vi "Raw Data Send Next Chunk.vi"(8 "error in (no error)":errorcluster, 10 "trimmed string":string, 11 "Network Info":T1 {"Last Comm Time" format="%<%H:%M:%S%3u\n%Y/%m/%d>T"; "Remote Port" format="%.0x"}) -> (0 "error out":errorcluster, 3 "Network Info Out":T1 {"Last Comm Time" format="%<%H:%M:%S%3u\n%Y/%m/%d>T"; "Remote Port" format="%.0x"})   [LabVIEW 2023]
doc: "Author: Scott Hannahs <sth@magnet.fsu.edu>\nCopyright 2018 Florida State University, All rights reserved."
uses:
  RT Controls/Network Info.ctl
  RT Controls/RT System Auth Level.ctl
  TCP Functions/TCP Write Length and Data (2D Array DBL).vi
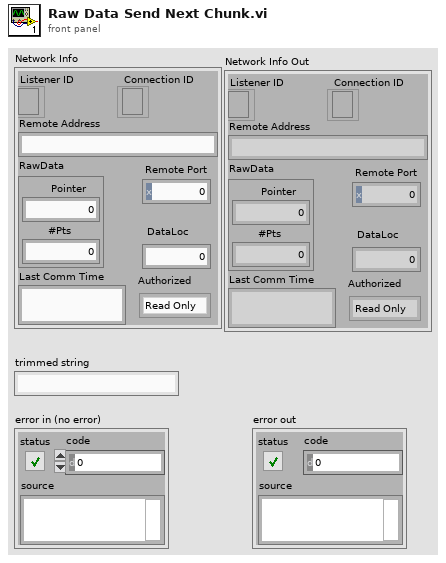
[diagram p1: front panel]
types:
  T1 = typedef "Network Info.ctl" = cluster{"Listener ID":refnum<k5>, "Connection ID":refnum<k5>, "Remote Address":string, "Remote Port":u16, "DataLoc":u32, "RawData":cluster{"#Pts":u32, "Pointer":u32}, "Last Comm Time":timestamp, "Authorized":T2}
  T2 = typedef "RT System Auth Level.ctl" = enum16{"Read Only", "Operator", "Admin"}
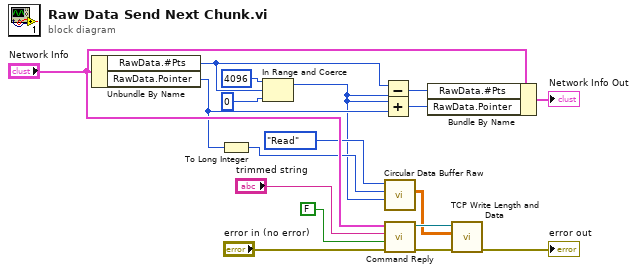
[diagram p0: block diagram]
diagram:
  n1 = Unbundle By Name("Network Info") -> ("RawData.#Pts"=w17:u32, "RawData.Pointer"=w6:u32)
  n2 = To Long Integer(number=w6) -> (32bit integer=w3:i32)
  n3 = In Range and Coerce(upper limit=u32 4096 ("y"), x=w17, lower limit=u32 0) -> (coerced(x)=w2:u32)  [unwired: 1 out]
  n4 = Subtract(x=w17, y=w2) -> (x-y=w8:u32)
  n5 = Add(x=w2, y=w6) -> (x+y=w7:u32)
  n6 = call "Circular Data Buffer Raw.vi"("Read Size"=w2, "Read Location"=w3, "Enum"=enum16{"Initialize", "Write", "Read", "Clear"}."Read" ("Action")) -> ("Data Out"=w1:dbl[][])  [unwired: 6 in, 2 out]
  n7 = call "Command Reply.vi"("Error In"="error in (no error)", "Error?"=FALSE, "String"="trimmed string", "Network Info"="Network Info") -> ("error out"=w16:errorcluster, "TCP Network Connection out"=w15:refnum<k5>)  [unwired: 6 in]
  n8 = Bundle By Name(cluster="Network Info", "RawData.#Pts"=w8, "RawData.Pointer"=w7) -> (→"Network Info Out":T1)
  n9 = call-poly "TCP Write Length and Data.vi"("Error In"=w16, "Data"=w1, "connection ID"=w15) -> ("Error Out"=→"error out":errorcluster)  [unwired: 7 in, 1 out]
